vi "XPS wait for acq.vi"(8 "error in (no error)":errorcluster) -> (0 "error out":errorcluster)   [LabVIEW 2020]
uses:
  shared/stop FGV control.ctl
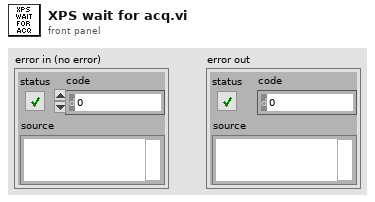
[diagram p1: front panel]
types:
  T1 = typedef "stop FGV control.ctl" = enum16{"Clear", "Write", "Read"}
  T2 = typedef "XPS Acquire FGV.ctl" = cluster{"busy":bool, "positions":dbl[]}
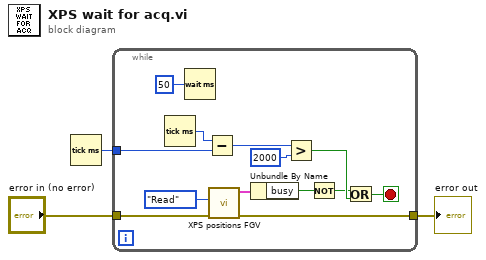
[diagram p0: block diagram]
diagram:
  n1 = Tick Count (ms)() -> (millisecond timer value=w3:u32)
  n2 = while {
    tunnel: "error in (no error)" -> [w12]
    tunnel: [w11] -> w2
    tunnel: w3 -> [w9]
    stop <- w4 stop-if-true
    n3 = Tick Count (ms)() -> (millisecond timer value=w10:u32)
    n4 = Wait (ms)(milliseconds to wait=u32 50) -> ()  [unwired: 1 out]
    n5 = Subtract(x=w10, y=w9) -> (x-y=w8:u32)
    n6 = call "XPS positions FGV.vi"("error in"=w12, "Function"=stop_FGV_control."Read") -> ("error out"=w11:errorcluster, "Acq Data out"=w15:T2)  [unwired: 8 in]
    n7 = Unbundle By Name(w15) -> ("busy"=w14:bool)
    n8 = Greater?(x=w8, y=u32 2000) -> (0:w6:bool)
    n9 = Not(x=w14) -> (.not. x?=w5:bool)
    n10 = Or(x=w5, y=w6) -> (x .or. y?=w4:bool)
  }
  "error out" <- w2
